vi "Array of Variants to Array Variant.vi"(8 "error in (no error)":errorcluster, 11 "[Variant]":variant[](array[variant])) -> (0 "error out":errorcluster, 3 "Array Variant":variant)   [LabVIEW 2018, in "TwinCAT ADS.lvclass"]
uses:
  TwinCAT ADS.lvclass
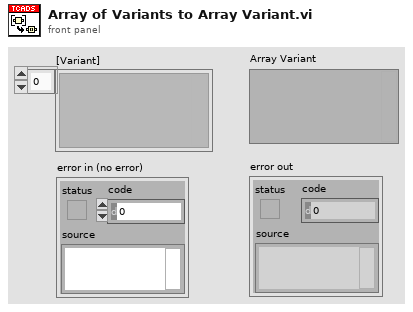
[diagram p1: front panel]
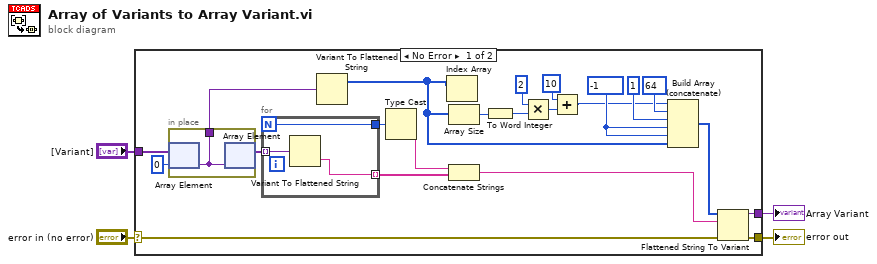
[diagram p0: block diagram]
diagram:
  n1 = case shown="No Error" "error in (no error)" {
    selector: "error in (no error)" -> [w20 w31]
    tunnel: [w19 w31] -> w3
    tunnel: "[Variant]" -> [w15 _]
    tunnel: [w18 _] -> w2
    frame No Error {
      w21 = i16 -1
      n2 = in-place {
        in-place-border: [w27] -> w12
        n3 = in-place-array #1(w15, 0) -> (w27:variant)
        n4 = in-place-array #1(w27) -> (w14:variant[])  [unwired: 1 out]
      }
      n5 = for {
        N -> [w30]
        tunnel: w14 -> [w29] mode=indexing
        tunnel: [w28] -> w26 mode=indexing
        tunnel: [w30] -> w16
        n6 = Variant To Flattened String(Variant=w29) -> (data string=w28:string)  [unwired: 1 out]
      }
      n7 = Variant To Flattened String(Variant=w12) -> (1:w9:i16[])  [unwired: 1 out]
      n8 = Type Cast(x=w16) -> (*(type *) &x=w25:string)  [unwired: 1 in]
      n9 = Index Array(array=w9) -> ()  [unwired: 1 in, 1 out]
      n10 = Array Size(array=w9) -> (size(s)=w24:i32)
      n11 = Concatenate Strings(w25, w26) -> (w17:string)
      n12 = To Word Integer(number=w24) -> (16bit integer=w6:i16)
      n13 = Multiply(x=i16 2, y=w6) -> (x*y=w8:i16)
      n14 = Add(x=i16 10, y=w8) -> (x+y=w10:i16)
      n15 = Build Array (concatenate)(w10, i16 64, i16 1 ("element"), w21, w21, w9) -> (w7:i16[])
      n16 = Flattened String To Variant(4:w20, 6:w17, 7:w7) -> (0:w19:errorcluster, 3:w18:variant)
    }
    frame Error {
    }
  }
  "error out" <- w3
  "Array Variant" <- w2
